vi "BW Create DB.vi"(9 "String":string="DROP TABLE IF EXISTS album;\nDROP TABLE IF EXISTS artist;\n\nCREATE TABLE artist (\n  id INTEGER PRIMARY KEY,\n  name TEXT\n);\n\nCREATE TABLE album (\n  id INTEGER PRIMARY KEY,\n  name TEXT,\n  artistid INTEGER\n);\n\nINSERT INTO artist VALUES\n(1, 'Richard Wagner'),\n(2, 'Ludwig van Beethoven');\n\nINSERT INTO album VALUES\n(NULL, 'Das Rheingold', 1),\n(NULL, 'Die Walkure', 1),\n(NULL, 'Siegfried', 1),\n(NULL, 'Gotterdammerung', 1),\n(NULL, 'Symphony No 5', 2),\n(NULL, 'Symphony No 9', 2);") -> (0 "error out":errorcluster)   [LabVIEW 2017, in "Beltwatch SQLite.lvlib"]
doc: "Drops any existing data from the test database and sets up tables for use in the project examples."
uses:
  <vilib>/drjdpowell/SQLite Library/SQL Connection/Open (string).vi
  Common64/Database/SQ Lite/SQ Lite Globals.vi
  <vilib>/drjdpowell/SQLite Library/SQL Connection/Connection.lvclass
  Beltwatch/BeltWatch 4-2-2-5/Database/Beltwatch SQLite.lvlib
panel:
  # "Drops any existing data from the test database and sets up tables for use in the project examples."
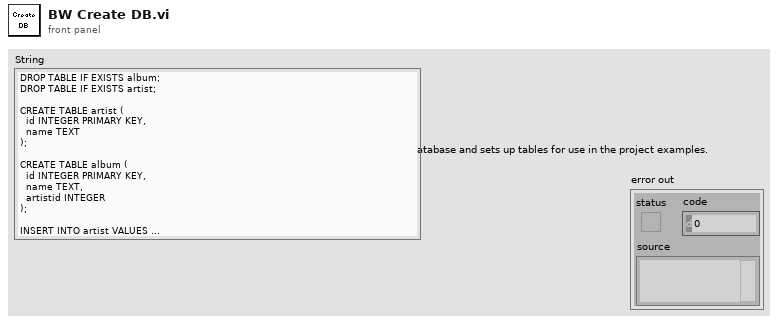
[diagram p1: front panel]
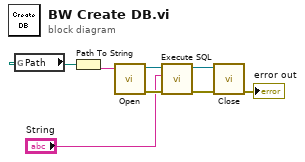
[diagram p0: block diagram]
diagram:
  n1 = global read "SQ Lite Globals.vi" "Path"() -> (w1:path)
  n2 = Path To String(path=w1) -> (string=w2:string)
  n3 = call-poly <vilib>:"Open.vi"("db file"=w2) -> ("error out"=w7:errorcluster, "SQLite Connection"=w8:refnum<class "Connection.lvclass">)  [unwired: 9 in]
  n4 = call <vilib>:"Execute SQL.vi"("error in (no error)"=w7, "SQL"="String", "SQLite Connection in"=w8) -> ("error out"=w3:errorcluster, "SQLite Connection"=w4:refnum<class "Connection.lvclass">)  [unwired: 5 in, 2 out]
  n5 = call-dynamic "Close.vi"("error in (no error)"=w3, "SQLite Connection in"=w4) -> ("error out"=→"error out":errorcluster)  [unwired: 9 in]
